vi "GasMeter3.vi"() -> ()   [LabVIEW 2012]
uses:
  <vilib>/DAQmx/read.llb/DAQmx Read (Analog 1D DBL NChan 1Samp).vi
panel:
  out "ANSI Placeholder 3":dbl
  out "Start Time ANSI 3":dbl
  out "ANSI Placeholder 2":dbl
  out "Start Time ANSI 2":dbl
  in  "Start ANSI 3":bool
  in  "HeatingValueLP 3":dbl=2450.0 min=2400.0 max=2600.0 step=5.0
  out "CF/HR 3":dbl format="%#_2g"
  out "HV 3":dbl
  out "Meter ID 3":dbl
  out "Gas 3":string
  in  "HeatingValueLP 2":dbl=2450.0 min=2400.0 max=2600.0 step=5.0
  in  "HeatingValueNG 2":dbl=990.0 min=990.0 max=1025.0 step=1.0
  out "Meter 6 Present":bool
  out "Meter 5 Present":bool
  out "Meter 4 Present":bool
  out "Meter 3 Present":bool
  out "Meter 2 Present":bool
  out "Meter 1 Present":bool
  out "Meter Type 6":string
  out "Meter Type 2":string
  out "Meter Type 4":string
  out "Meter Type 5":string
  out "Meter Type 3":string
  out "Meter Type 1":string
  out "Meter 6 Size":dbl
  out "Meter 5 Size":dbl
  out "Meter 4 Size":dbl
  out "Meter 3 Size":dbl
  out "Meter 2 Size":dbl
  out "Meter 1 Size":dbl
  out "ANSI Placeholder":dbl
  out "Start Time ANSI":dbl
  in  "Start ANSI":bool
  out "ANSI Average (BTU/hr)":dbl format="%#_5g"
  out "30 Second Average (BTU/hr)":dbl format="%#_5g"
  out "15 Second Average (BTU/hr)":dbl format="%#_5g"
  out "Reference6":dbl
  out "Reference5":dbl
  out "Reference4":dbl
  out "Reference3":dbl
  out "Reference2":dbl
  out "Reference1":dbl
  out "Time":dbl
  out "Num Record":dbl
  in  "HeatingValueLP":dbl=2450.0 min=2400.0 max=2600.0 step=5.0
  out "Output 6":dbl min=0.0 max=5.0 step=0.01
  out "Output 5":dbl min=0.0 max=5.0 step=0.01
  out "Output 4":dbl min=0.0 max=5.0 step=0.01
  out "Output 3":dbl min=0.0 max=5.0 step=0.01
  out "Output 2":dbl min=0.0 max=5.0 step=0.01
  out "Output 1":dbl min=0.0 max=5.0 step=0.01
  out "Signal":bool
  in  "Record":bool
  out "File Path":path
  out "CF/HR":dbl format="%#_2g"
  out "HV":dbl
  in  "HeatingValueNG":dbl=990.0 min=990.0 max=1025.0 step=1.0
  out "Meter ID":dbl
  out "Gas":string
  out "DisplayChart":cluster{"Flow Rate":dbl}(graph)
  out "Flow Rate":dbl format="%#_5g"
  # "STATION 1"
  # "STATION 3"
  # "Heating Value"
  # "Heating Value"
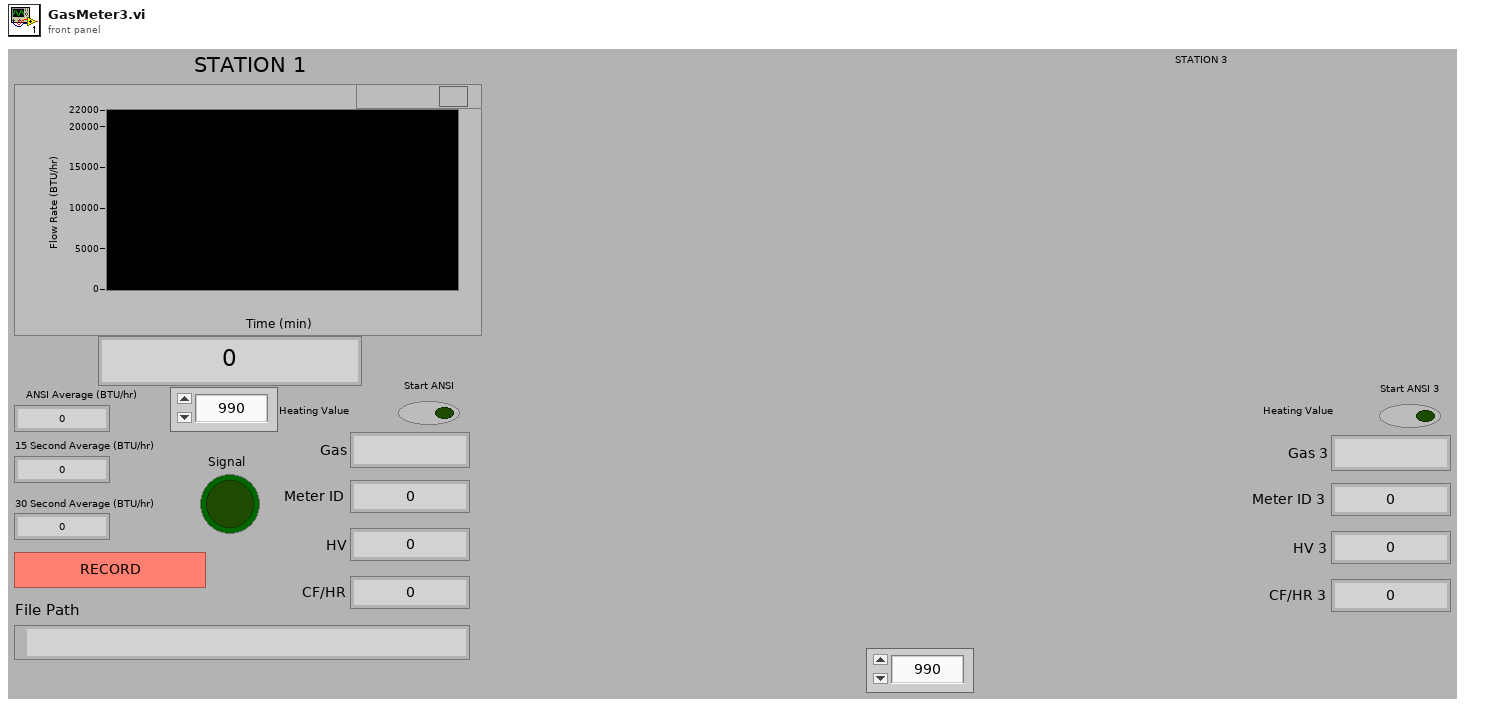
[diagram p1: front panel]
types:
  T1 = enum16{"open", "replace", "create", "open or create", "replace or create", "replace or create with confirmation"}
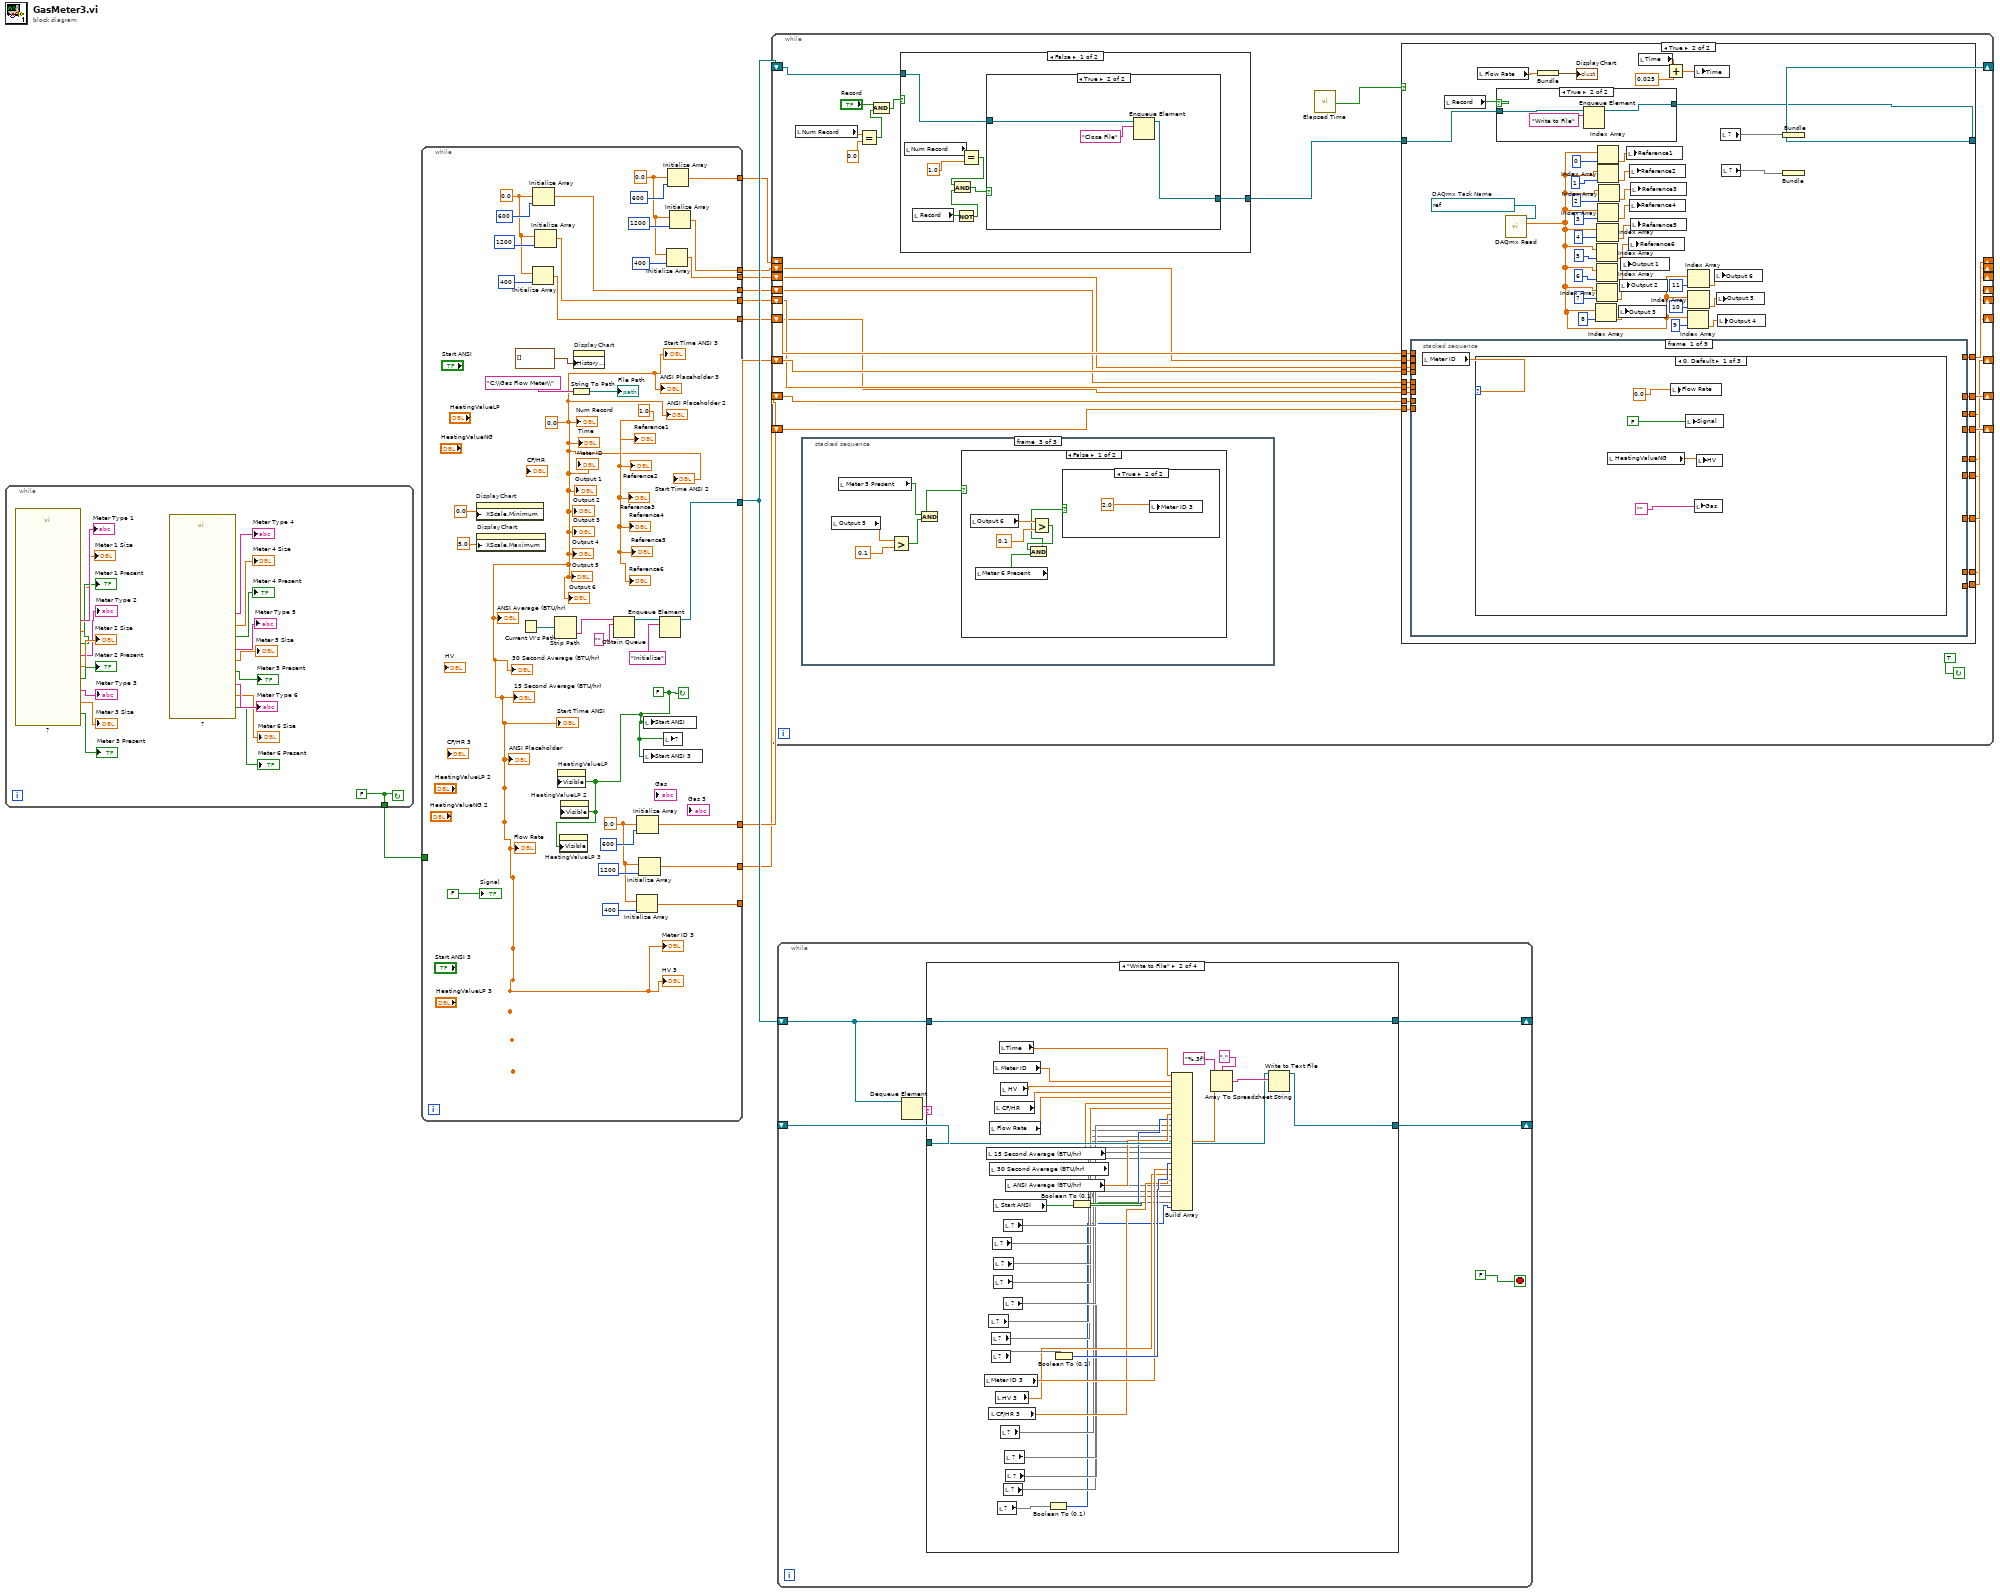
[diagram p0: block diagram]
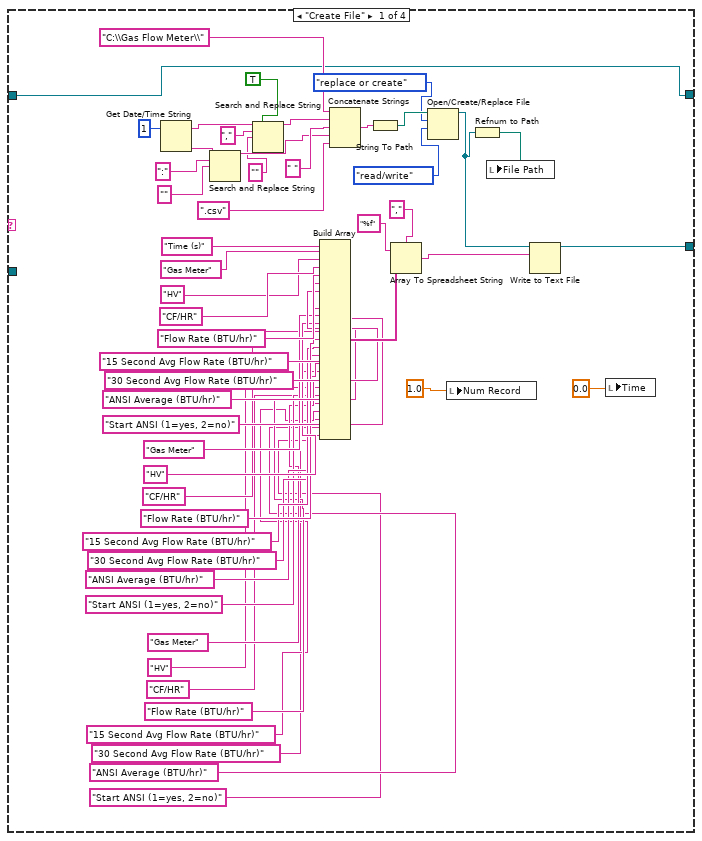
[diagram p2: hidden frame]
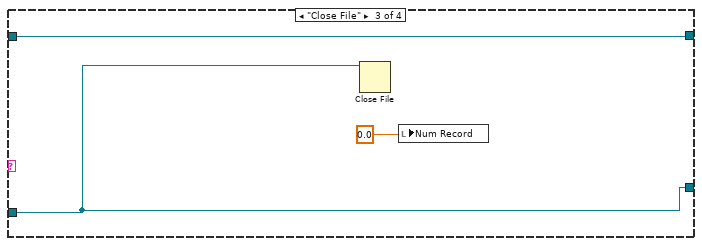
[diagram p3: hidden frame]
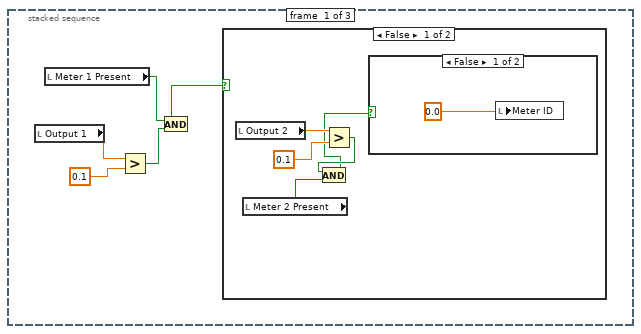
[diagram p5: hidden frame]
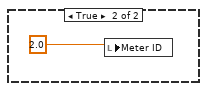
[diagram p6: hidden frame]
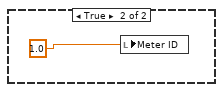
[diagram p7: hidden frame]
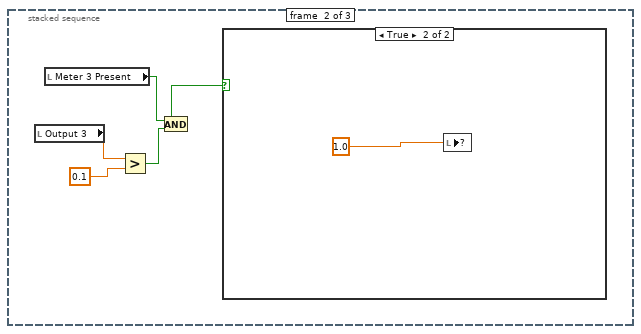
[diagram p8: hidden frame]
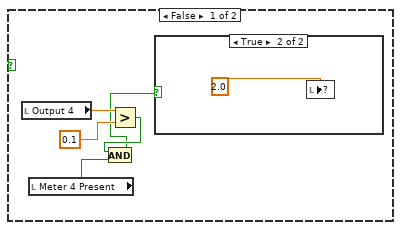
[diagram p9: hidden frame]
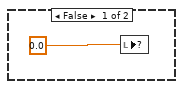
[diagram p10: hidden frame]
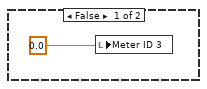
[diagram p11: hidden frame]
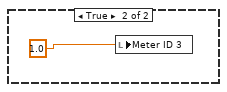
[diagram p12: hidden frame]
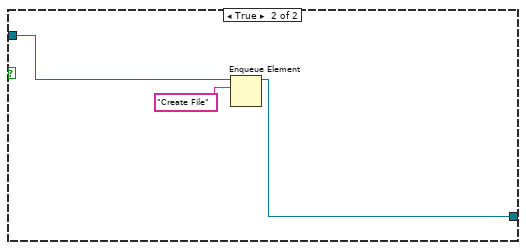
[diagram p14: hidden frame]
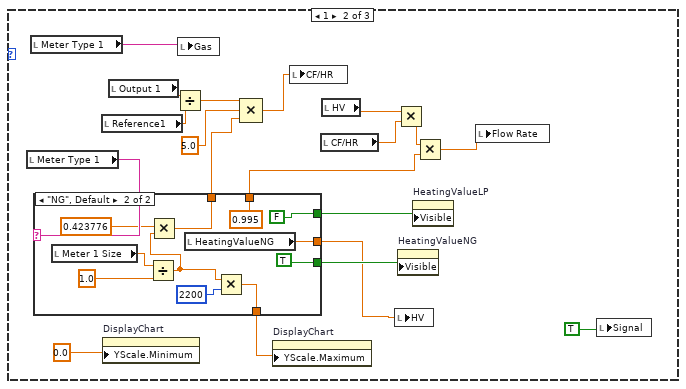
[diagram p16: hidden frame]
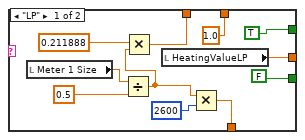
[diagram p17: hidden frame]
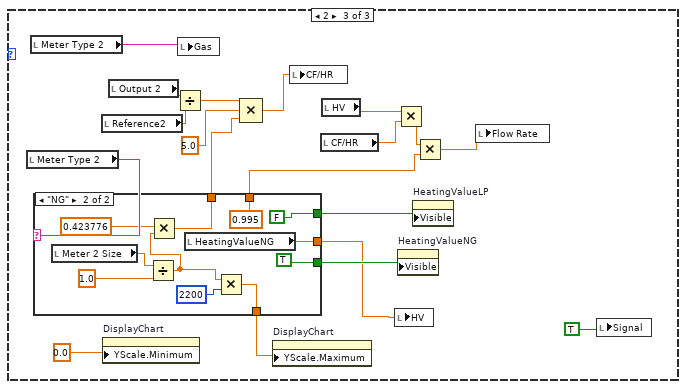
[diagram p18: hidden frame]
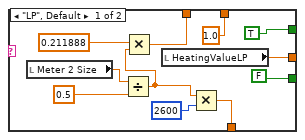
[diagram p19: hidden frame]
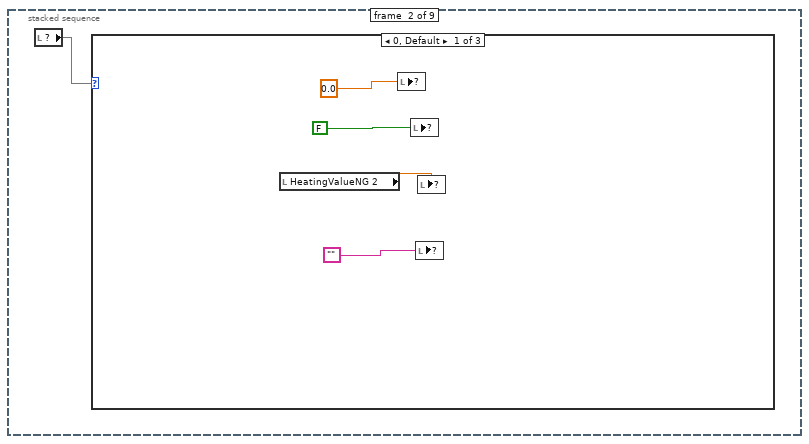
[diagram p20: hidden frame]
diagram:
  n1 = while {
    tunnel: [w29] -> w7
    stop <- w29 continue-if-true
    w29 = FALSE
    n2 = call "?"() -> ("Meter 3 Present?"=→"Meter 3 Present":bool, "Meter Size 3 (SLPM)"=→"Meter 3 Size":dbl, "Meter Type 3 (LP/NG)"=→"Meter Type 3":string, "Meter 2 Present?"=→"Meter 2 Present":bool, "Meter Size 2 (SLPM)"=→"Meter 2 Size":dbl, "Meter Type 2 (LP/NG)"=→"Meter Type 2":string, "Meter 1 Present?"=→"Meter 1 Present":bool, "Meter Size 1 (SLPM)"=→"Meter 1 Size":dbl, "Meter Type 1 (LP/NG)"=→"Meter Type 1":string)  [unwired: 9 in, 2 out]
    n3 = call "?"() -> ("Meter 6 Present?"=→"Meter 6 Present":bool, "Meter Size 6 (SLPM)"=→"Meter 6 Size":dbl, "Meter Type 6 (LP/NG)"=→"Meter Type 6":string, "Meter 5 Present?"=→"Meter 5 Present":bool, "Meter Size 5 (SLPM)"=→"Meter 5 Size":dbl, "Meter Type 5 (LP/NG)"=→"Meter Type 5":string, "Meter 4 Present?"=→"Meter 4 Present":bool, "Meter Size 4 (SLPM)"=→"Meter 4 Size":dbl, "Meter Type 4 (LP/NG)"=→"Meter Type 4":string)  [unwired: 9 in, 2 out]
  }
  n4 = while {
    tunnel: [w59] -> w11
    tunnel: [w55] -> w10
    tunnel: [w54] -> w9
    tunnel: [w51] -> w8
    tunnel: w7 -> [_]
    tunnel: [w46] -> w6
    tunnel: [w45] -> w5
    tunnel: [w44] -> w4
    tunnel: [w39] -> w3
    tunnel: [w38] -> w2
    tunnel: [w37] -> w1
    stop <- w34 continue-if-true
    w41 = 0.0
    w48 = 0.0
    w53 = 0.0
    w58 = 1.0
    w35 = 0.0
    w34 = FALSE
    n5 = property on="DisplayChart" class="WFChart (strict)"("XScale.Minimum"=0.0) -> ()  [unwired: 2 in, 2 out]
    n6 = property on="DisplayChart" class="WFChart (strict)"("XScale.Maximum"=5.0) -> ()  [unwired: 2 in, 2 out]
    n7 = Current VI's Path() -> (path=w64:path)
    n8 = Initialize Array(w41, 400) -> (w37:dbl[])
    n9 = Initialize Array(w41, 600) -> (w39:dbl[])
    n10 = Initialize Array(w41, 1200) -> (w38:dbl[])
    n11 = Strip Path(path=w64) -> (name=w62:string)  [unwired: 1 out]
    n12 = property on="HeatingValueLP" class="DigNum (strict)"("Visible"=w34) -> ()  [unwired: 2 in, 2 out]
    n13 = property on="HeatingValueLP 3" class="DigNum (strict)"("Visible"=w34) -> ()  [unwired: 2 in, 2 out]
    n14 = property on="HeatingValueLP 2" class="DigNum (strict)"("Visible"=w34) -> ()  [unwired: 2 in, 2 out]
    n15 = String To Path(string="C:\\Gas Flow Meter\\") -> (path=→"File Path":path)
    n16 = property on="DisplayChart" class="WFChart (strict)"("History Data"=cluster{"[0]":dbl}[] []) -> ()  [unwired: 2 in, 2 out]
    n17 = Obtain Queue(name (unnamed)=w62, element data type="") -> (queue out=w60:refnum<queue>)  [unwired: 3 in, 2 out]
    n18 = Initialize Array(w53, 400) -> (w51:dbl[])
    n19 = Initialize Array(w53, 600) -> (w55:dbl[])
    n20 = Initialize Array(w53, 1200) -> (w54:dbl[])
    n21 = local write "Start ANSI"(w34) -> ()
    n22 = local write "Start ANSI 3"(w34) -> ()
    n23 = Enqueue Element(queue=w60, element="Initialize") -> (queue out=w59:refnum<queue>)  [unwired: 2 in, 2 out]
    n24 = local write item#-1(w34) -> ()
    n25 = Initialize Array(w48, 400) -> (w44:dbl[])
    n26 = Initialize Array(w48, 600) -> (w46:dbl[])
    n27 = Initialize Array(w48, 1200) -> (w45:dbl[])
    "Num Record" <- w35
    "Time" <- w35
    "Meter ID" <- w35
    "Output 1" <- w35
    "Output 2" <- w35
    "Output 3" <- w35
    "Output 4" <- w35
    "Output 5" <- w35
    "Output 6" <- w35
    "Reference1" <- w58
    "Reference2" <- w58
    "Reference3" <- w58
    "Reference4" <- w58
    "Reference5" <- w58
    "Reference6" <- w58
    "30 Second Average (BTU/hr)" <- w35
    "15 Second Average (BTU/hr)" <- w35
    "ANSI Average (BTU/hr)" <- w35
    "Start Time ANSI" <- w35
    "ANSI Placeholder" <- w35
    "Flow Rate" <- w35
    "Signal" <- FALSE
    "Meter ID 3" <- w35
    "HV 3" <- w35
    "Start Time ANSI 3" <- w35
    "ANSI Placeholder 3" <- w35
    "ANSI Placeholder 2" <- w35
    "Start Time ANSI 2" <- w35
  }
  n28 = while {
    shift-right: [w92] -> _
    shift-left: w11 -> [w85]
    shift-right: [w91] -> _
    shift-left: w10 -> [w89]
    shift-right: [w90] -> _
    shift-left: w9 -> [w88]
    shift-right: [w87] -> _
    shift-left: w8 -> [w86]
    shift-right: [w77] -> _
    shift-left: w6 -> [w78]
    shift-right: [w75] -> _
    shift-left: w5 -> [w76]
    shift-right: [w73] -> _
    shift-left: w4 -> [w74]
    shift-right: [w71] -> _
    shift-left: w3 -> [w72]
    shift-right: [w69] -> _
    shift-left: w2 -> [w70]
    shift-right: [w67] -> _
    shift-left: w1 -> [w68]
    stop <- TRUE continue-if-true
    n29 = local read "Num Record"() -> (w81:dbl)
    n30 = stacked-sequence {
      frame #0 {
        n31 = local read "Output 1"() -> (w99:dbl)
        n32 = local read "Meter 1 Present"() -> (w96:bool)
        n33 = Greater?(x=w99, y=0.1) -> (0:w97:bool)
        n34 = And(x=w96, y=w97) -> (x .and. y?=w95:bool)
        n35 = case shown="False" w95 {
          frame False {
            n36 = local read "Output 2"() -> (w103:dbl)
            n37 = local read "Meter 2 Present"() -> (w102:bool)
            n38 = Greater?(x=w103, y=0.1) -> (0:w101:bool)
            n39 = And(x=w101, y=w102) -> (x .and. y?=w100:bool)
            n40 = case shown="False" w100 {
              frame False {
                n41 = local write "Meter ID"(0.0) -> ()
              }
              frame True {
                n42 = local write "Meter ID"(2.0) -> ()
              }
            }
          }
          frame True {
            n43 = local write "Meter ID"(1.0) -> ()
          }
        }
      }
      frame #1 {
        n44 = local read "Output 3"() -> (w112:dbl)
        n45 = local read "Meter 3 Present"() -> (w109:bool)
        n46 = Greater?(x=w112, y=0.1) -> (0:w110:bool)
        n47 = And(x=w109, y=w110) -> (x .and. y?=w108:bool)
        n48 = case shown="True" w108 {
          frame False {
            n49 = local read "Output 4"() -> (w116:dbl)
            n50 = local read "Meter 4 Present"() -> (w115:bool)
            n51 = Greater?(x=w116, y=0.1) -> (0:w114:bool)
            n52 = And(x=w114, y=w115) -> (x .and. y?=w113:bool)
            n53 = case shown="True" w113 {
              frame False {
                n54 = local write item#-1(0.0) -> ()
              }
              frame True {
                n55 = local write item#-1(2.0) -> ()
              }
            }
          }
          frame True {
            n56 = local write item#-1(1.0) -> ()
          }
        }
      }
      frame #2 {
        n57 = local read "Output 5"() -> (w125:dbl)
        n58 = local read "Meter 5 Present"() -> (w122:bool)
        n59 = Greater?(x=w125, y=0.1) -> (0:w123:bool)
        n60 = And(x=w122, y=w123) -> (x .and. y?=w121:bool)
        n61 = case shown="False" w121 {
          frame False {
            n62 = local read "Output 6"() -> (w129:dbl)
            n63 = local read "Meter 6 Present"() -> (w128:bool)
            n64 = Greater?(x=w129, y=0.1) -> (0:w127:bool)
            n65 = And(x=w127, y=w128) -> (x .and. y?=w126:bool)
            n66 = case shown="True" w126 {
              frame False {
                n67 = local write "Meter ID 3"(0.0) -> ()
              }
              frame True {
                n68 = local write "Meter ID 3"(2.0) -> ()
              }
            }
          }
          frame True {
            n69 = local write "Meter ID 3"(1.0) -> ()
          }
        }
      }
    }
    n70 = Equal?(x=w81, y=0.0) -> (x = y?=w80:bool)
    n71 = And(x="Record", y=w80) -> (x .and. y?=w79:bool)
    n72 = case shown="False" w79 {
      tunnel: w85 -> [w139 w147]
      tunnel: [w138 w146] -> w84
      frame False {
        n73 = local read "Num Record"() -> (w141:dbl)
        n74 = local read "Record"() -> (w135:bool)
        n75 = Not(x=w135) -> (.not. x?=w134:bool)
        n76 = Equal?(x=w141, y=1.0) -> (x = y?=w137:bool)
        n77 = And(x=w137, y=w134) -> (x .and. y?=w136:bool)
        n78 = case shown="True" w136 {
          tunnel: w139 -> [w142 w144]
          tunnel: [w142 w143] -> w138
          frame False {
          }
          frame True {
            n79 = Enqueue Element(queue=w144, element="Close File") -> (queue out=w143:refnum<queue>)  [unwired: 2 in, 2 out]
          }
        }
      }
      frame True {
        n80 = Enqueue Element(queue=w147, element="Create File") -> (queue out=w146:refnum<queue>)  [unwired: 2 in, 2 out]
      }
    }
    n81 = call "Elapsed Time"() -> ("Time has Elapsed"=w93:bool)  [unwired: 12 in, 7 out]
    n82 = case shown="True" w93 {
      tunnel: w84 -> [w158 w208]
      tunnel: [w158 w207] -> w92
      tunnel: w89 -> [w157 w180]
      tunnel: w88 -> [w156 w179]
      tunnel: [w157 w178] -> w91
      tunnel: [w156 w177] -> w90
      tunnel: w86 -> [w155 w176]
      tunnel: [w155 w175] -> w87
      tunnel: w78 -> [w152 w174]
      tunnel: [w152 w173] -> w77
      tunnel: w76 -> [w153 w172]
      tunnel: [w153 w171] -> w75
      tunnel: w74 -> [w154 w170]
      tunnel: [w154 w169] -> w73
      tunnel: w72 -> [w151 w168]
      tunnel: [w151 w167] -> w71
      tunnel: w70 -> [w150 w166]
      tunnel: [w150 w165] -> w69
      tunnel: w68 -> [w149 w164]
      tunnel: [w149 w163] -> w67
      frame False {
      }
      frame True {
        w206 = refnum<k21> "ReadFlowMeterIn"  # DAQmx Task Name
        n83 = stacked-sequence {
          tunnel: w180 -> [_ _ _ w500 _ _ _ _ _]
          tunnel: w179 -> [_ _ _ w499 _ _ _ _ _]
          tunnel: [_ _ _ w494 _ _ _ _ _] -> w178
          tunnel: [_ _ _ w490 _ _ _ _ _] -> w177
          tunnel: w176 -> [_ _ _ w484 _ _ _ _ _]
          tunnel: [_ _ _ w481 _ _ _ _ _] -> w175
          tunnel: w174 -> [_ _ _ _ w523 _ _ _ _]
          tunnel: [_ _ _ _ w510 _ _ _ _] -> w173
          tunnel: w172 -> [_ _ _ _ w517 _ _ _ _]
          tunnel: [_ _ _ _ w509 _ _ _ _] -> w171
          tunnel: w170 -> [_ _ _ _ w515 _ _ _ _]
          tunnel: [_ _ _ _ w508 _ _ _ _] -> w169
          tunnel: w168 -> [_ _ _ _ _ w544 _ _ _]
          tunnel: [_ _ _ _ _ w542 _ _ _] -> w167
          tunnel: w166 -> [_ _ _ _ _ w541 _ _ _]
          tunnel: [_ _ _ _ _ w539 _ _ _] -> w165
          tunnel: w164 -> [_ _ _ _ _ w538 _ _ _]
          tunnel: [_ _ _ _ _ w536 _ _ _] -> w163
          frame #0 {
            n84 = local read "Meter ID"() -> (w215:dbl)
            n85 = case shown="0, Default" w215 {
              frame 0, Default {
                n86 = local read "HeatingValueNG"() -> (w219:dbl)
                n87 = local write "Flow Rate"(0.0) -> ()
                n88 = local write "Signal"(FALSE) -> ()
                n89 = local write "Gas"("") -> ()
                n90 = local write "HV"(w219) -> ()
              }
              frame 1 {
                n91 = local read "Meter Type 1"() -> (w228:string)
                n92 = local read "Meter Type 1"() -> (w222:string)
                n93 = case shown="\"NG\", Default" w228 {
                  tunnel: [w246 w257] -> w227
                  tunnel: [TRUE FALSE] -> w226
                  tunnel: [FALSE TRUE] -> w225
                  tunnel: [1.0 0.995] -> w224
                  tunnel: [w240 w251] -> w223
                  tunnel: [w239 w250] -> w221
                  frame "LP" {
                    n94 = local read "Meter 1 Size"() -> (w248:dbl)
                    n95 = Divide(x=w248, y=0.5) -> (x/y=w241:dbl)
                    n96 = Multiply(x=0.211888, y=w241) -> (x*y=w246:dbl)
                    n97 = local read "HeatingValueLP"() -> (w239:dbl)
                    n98 = Multiply(x=w241, y=2600) -> (x*y=w240:dbl)
                  }
                  frame "NG", Default {
                    n99 = local read "Meter 1 Size"() -> (w259:dbl)
                    n100 = Divide(x=w259, y=1.0) -> (x/y=w252:dbl)
                    n101 = Multiply(x=0.423776, y=w252) -> (x*y=w257:dbl)
                    n102 = local read "HeatingValueNG"() -> (w250:dbl)
                    n103 = Multiply(x=w252, y=2200) -> (x*y=w251:dbl)
                  }
                }
                n104 = local read "Reference1"() -> (w232:dbl)
                n105 = property on="DisplayChart" class="WFChart (strict)"("YScale.Minimum"=0.0) -> ()  [unwired: 2 in, 2 out]
                n106 = local read "Output 1"() -> (w233:dbl)
                n107 = Divide(x=w233, y=w232) -> (x/y=w230:dbl)
                n108 = local write "Gas"(w222) -> ()
                n109 = Compound Arithmetic op=MULTIPLY(w230, 5.0, w227) -> (w220:dbl)
                n110 = property on="DisplayChart" class="WFChart (strict)"("YScale.Maximum"=w223) -> ()  [unwired: 2 in, 2 out]
                n111 = local write "CF/HR"(w220) -> ()
                n112 = local read "CF/HR"() -> (w235:dbl)
                n113 = local read "HV"() -> (w234:dbl)
                n114 = local write "HV"(w221) -> ()
                n115 = Multiply(x=w234, y=w235) -> (x*y=w236:dbl)
                n116 = property on="HeatingValueNG" class="DigNum (strict)"("Visible"=w225) -> ()  [unwired: 2 in, 2 out]
                n117 = property on="HeatingValueLP" class="DigNum (strict)"("Visible"=w226) -> ()  [unwired: 2 in, 2 out]
                n118 = Multiply(x=w236, y=w224) -> (x*y=w237:dbl)
                n119 = local write "Flow Rate"(w237) -> ()
                n120 = local write "Signal"(TRUE) -> ()
              }
              frame 2 {
                n121 = local read "Meter Type 2"() -> (w269:string)
                n122 = local read "Meter Type 2"() -> (w263:string)
                n123 = case shown="\"NG\"" w269 {
                  tunnel: [w287 w298] -> w268
                  tunnel: [TRUE FALSE] -> w267
                  tunnel: [FALSE TRUE] -> w266
                  tunnel: [1.0 0.995] -> w265
                  tunnel: [w281 w292] -> w264
                  tunnel: [w280 w291] -> w262
                  frame "LP", Default {
                    n124 = local read "Meter 2 Size"() -> (w289:dbl)
                    n125 = Divide(x=w289, y=0.5) -> (x/y=w282:dbl)
                    n126 = Multiply(x=0.211888, y=w282) -> (x*y=w287:dbl)
                    n127 = local read "HeatingValueLP"() -> (w280:dbl)
                    n128 = Multiply(x=w282, y=2600) -> (x*y=w281:dbl)
                  }
                  frame "NG" {
                    n129 = local read "Meter 2 Size"() -> (w300:dbl)
                    n130 = Divide(x=w300, y=1.0) -> (x/y=w293:dbl)
                    n131 = Multiply(x=0.423776, y=w293) -> (x*y=w298:dbl)
                    n132 = local read "HeatingValueNG"() -> (w291:dbl)
                    n133 = Multiply(x=w293, y=2200) -> (x*y=w292:dbl)
                  }
                }
                n134 = local read "Reference2"() -> (w273:dbl)
                n135 = property on="DisplayChart" class="WFChart (strict)"("YScale.Minimum"=0.0) -> ()  [unwired: 2 in, 2 out]
                n136 = local read "Output 2"() -> (w274:dbl)
                n137 = Divide(x=w274, y=w273) -> (x/y=w271:dbl)
                n138 = local write "Gas"(w263) -> ()
                n139 = Compound Arithmetic op=MULTIPLY(w271, 5.0, w268) -> (w261:dbl)
                n140 = property on="DisplayChart" class="WFChart (strict)"("YScale.Maximum"=w264) -> ()  [unwired: 2 in, 2 out]
                n141 = local write "CF/HR"(w261) -> ()
                n142 = local read "CF/HR"() -> (w276:dbl)
                n143 = local read "HV"() -> (w275:dbl)
                n144 = local write "HV"(w262) -> ()
                n145 = Multiply(x=w275, y=w276) -> (x*y=w277:dbl)
                n146 = property on="HeatingValueNG" class="DigNum (strict)"("Visible"=w266) -> ()  [unwired: 2 in, 2 out]
                n147 = property on="HeatingValueLP" class="DigNum (strict)"("Visible"=w267) -> ()  [unwired: 2 in, 2 out]
                n148 = Multiply(x=w277, y=w265) -> (x*y=w278:dbl)
                n149 = local write "Flow Rate"(w278) -> ()
                n150 = local write "Signal"(TRUE) -> ()
              }
            }
          }
          frame #1 {
            n151 = local read item#-1() -> (w302)
            n152 = case shown="0, Default" w302 {
              frame 0, Default {
                n153 = local read "HeatingValueNG 2"() -> (w306:dbl)
                n154 = local write item#-1(0.0) -> ()
                n155 = local write item#-1(FALSE) -> ()
                n156 = local write item#-1("") -> ()
                n157 = local write item#-1(w306) -> ()
              }
              frame 1 {
                w316 = 0.0
                n158 = local read "Meter Type 3"() -> (w315:string)
                n159 = local read "Meter Type 3"() -> (w309:string)
                n160 = case shown="\"LP\"" w315 {
                  tunnel: [w333 w344] -> w314
                  tunnel: [TRUE FALSE] -> w313
                  tunnel: [FALSE TRUE] -> w312
                  tunnel: [1.0 0.995] -> w311
                  tunnel: [w327 w338] -> w310
                  tunnel: [w326 w337] -> w308
                  frame "LP" {
                    n161 = local read "Meter 3 Size"() -> (w335:dbl)
                    n162 = Divide(x=w335, y=0.5) -> (x/y=w328:dbl)
                    n163 = Multiply(x=0.211888, y=w328) -> (x*y=w333:dbl)
                    n164 = local read "HeatingValueLP 2"() -> (w326:dbl)
                    n165 = Multiply(x=w328, y=2600) -> (x*y=w327:dbl)
                  }
                  frame "NG", Default {
                    n166 = local read "Meter 3 Size"() -> (w346:dbl)
                    n167 = Divide(x=w346, y=1.0) -> (x/y=w339:dbl)
                    n168 = Multiply(x=0.423776, y=w339) -> (x*y=w344:dbl)
                    n169 = local read "HeatingValueNG 2"() -> (w337:dbl)
                    n170 = Multiply(x=w339, y=2200) -> (x*y=w338:dbl)
                  }
                }
                n171 = local read "Reference3"() -> (w319:dbl)
                n172 = local read "Output 3"() -> (w320:dbl)
                n173 = Divide(x=w320, y=w319) -> (x/y=w317:dbl)
                n174 = local write item#-1(w309) -> ()
                n175 = Compound Arithmetic op=MULTIPLY(w317, 5.0, w314) -> (w307:dbl)
                n176 = local write item#-1(w307) -> ()
                n177 = local read item#-1() -> (w321)
                n178 = local read item#-1() -> (w322)
                n179 = Multiply(x=w321, y=w322) -> (x*y=w323:dbl)
                n180 = property on="HeatingValueNG 2" class="DigNum (strict)"("Visible"=w312) -> ()  [unwired: 2 in, 2 out]
                n181 = local write item#-1(w308) -> ()
                n182 = property on="HeatingValueLP 2" class="DigNum (strict)"("Visible"=w313) -> ()  [unwired: 2 in, 2 out]
                n183 = Multiply(x=w323, y=w311) -> (x*y=w324:dbl)
                n184 = local write item#-1(w324) -> ()
                n185 = local write item#-1(TRUE) -> ()
              }
              frame 2 {
                w357 = 0.0
                n186 = local read "Meter Type 4"() -> (w356:string)
                n187 = local read "Meter Type 4"() -> (w350:string)
                n188 = case shown="\"NG\", Default" w356 {
                  tunnel: [w374 w385] -> w355
                  tunnel: [TRUE FALSE] -> w354
                  tunnel: [FALSE TRUE] -> w353
                  tunnel: [1.0 0.995] -> w352
                  tunnel: [w368 w379] -> w351
                  tunnel: [w367 w378] -> w349
                  frame "LP" {
                    n189 = local read "Meter 4 Size"() -> (w376:dbl)
                    n190 = Divide(x=w376, y=0.5) -> (x/y=w369:dbl)
                    n191 = Multiply(x=0.211888, y=w369) -> (x*y=w374:dbl)
                    n192 = local read "HeatingValueLP 2"() -> (w367:dbl)
                    n193 = Multiply(x=w369, y=2600) -> (x*y=w368:dbl)
                  }
                  frame "NG", Default {
                    n194 = local read "Meter 4 Size"() -> (w387:dbl)
                    n195 = Divide(x=w387, y=1.0) -> (x/y=w380:dbl)
                    n196 = Multiply(x=0.423776, y=w380) -> (x*y=w385:dbl)
                    n197 = local read "HeatingValueNG 2"() -> (w378:dbl)
                    n198 = Multiply(x=w380, y=2200) -> (x*y=w379:dbl)
                  }
                }
                n199 = local read "Reference4"() -> (w360:dbl)
                n200 = local read "Output 4"() -> (w361:dbl)
                n201 = Divide(x=w361, y=w360) -> (x/y=w358:dbl)
                n202 = local write item#-1(w350) -> ()
                n203 = Compound Arithmetic op=MULTIPLY(w358, 5.0, w355) -> (w348:dbl)
                n204 = local write item#-1(w348) -> ()
                n205 = local read item#-1() -> (w362)
                n206 = local read item#-1() -> (w363)
                n207 = Multiply(x=w362, y=w363) -> (x*y=w364:dbl)
                n208 = property on="HeatingValueNG 2" class="DigNum (strict)"("Visible"=w353) -> ()  [unwired: 2 in, 2 out]
                n209 = local write item#-1(w349) -> ()
                n210 = property on="HeatingValueLP 2" class="DigNum (strict)"("Visible"=w354) -> ()  [unwired: 2 in, 2 out]
                n211 = Multiply(x=w364, y=w352) -> (x*y=w365:dbl)
                n212 = local write item#-1(w365) -> ()
                n213 = local write item#-1(TRUE) -> ()
              }
            }
          }
          frame #2 {
            n214 = local read "Meter ID 3"() -> (w389:dbl)
            n215 = case shown="0, Default" w389 {
              frame 0, Default {
                n216 = local read item#-1() -> (w393)
                n217 = local write item#-1(0.0) -> ()
                n218 = local write "Gas 3"("") -> ()
                n219 = local write "HV 3"(w393) -> ()
                n220 = local write item#-1(FALSE) -> ()
              }
              frame 1 {
                w403 = 0.0
                n221 = local read "Meter Type 5"() -> (w402:string)
                n222 = local read "Meter Type 5"() -> (w396:string)
                n223 = case shown="\"LP\"" w402 {
                  tunnel: [w420 w431] -> w401
                  tunnel: [TRUE FALSE] -> w400
                  tunnel: [FALSE TRUE] -> w399
                  tunnel: [1.0 0.995] -> w398
                  tunnel: [w414 w425] -> w397
                  tunnel: [w413 w424] -> w395
                  frame "LP" {
                    n224 = local read "Meter 5 Size"() -> (w422:dbl)
                    n225 = Divide(x=w422, y=0.5) -> (x/y=w415:dbl)
                    n226 = Multiply(x=0.211888, y=w415) -> (x*y=w420:dbl)
                    n227 = local read "HeatingValueLP 3"() -> (w413:dbl)
                    n228 = Multiply(x=w415, y=2600) -> (x*y=w414:dbl)
                  }
                  frame "NG", Default {
                    n229 = local read "Meter 5 Size"() -> (w433:dbl)
                    n230 = Divide(x=w433, y=1.0) -> (x/y=w426:dbl)
                    n231 = Multiply(x=0.423776, y=w426) -> (x*y=w431:dbl)
                    n232 = Multiply(x=w426, y=2200) -> (x*y=w425:dbl)
                    n233 = local read item#-1() -> (w424)
                  }
                }
                n234 = local read "Reference5"() -> (w406:dbl)
                n235 = local read "Output 5"() -> (w407:dbl)
                n236 = local write "Gas 3"(w396) -> ()
                n237 = Divide(x=w407, y=w406) -> (x/y=w404:dbl)
                n238 = Compound Arithmetic op=MULTIPLY(w404, 5.0, w401) -> (w394:dbl)
                n239 = local write "CF/HR 3"(w394) -> ()
                n240 = local read "CF/HR 3"() -> (w409:dbl)
                n241 = local read "HV 3"() -> (w408:dbl)
                n242 = local write "HV 3"(w395) -> ()
                n243 = Multiply(x=w408, y=w409) -> (x*y=w410:dbl)
                n244 = property on="HeatingValueLP 3" class="DigNum (strict)"("Visible"=w400) -> ()  [unwired: 2 in, 2 out]
                n245 = Multiply(x=w410, y=w398) -> (x*y=w411:dbl)
                n246 = local write item#-1(w411) -> ()
                n247 = local write item#-1(TRUE) -> ()
              }
              frame 2 {
                w444 = 0.0
                n248 = local read "Meter Type 6"() -> (w443:string)
                n249 = local read "Meter Type 6"() -> (w437:string)
                n250 = case shown="\"NG\", Default" w443 {
                  tunnel: [w461 w472] -> w442
                  tunnel: [TRUE FALSE] -> w441
                  tunnel: [FALSE TRUE] -> w440
                  tunnel: [1.0 0.995] -> w439
                  tunnel: [w455 w466] -> w438
                  tunnel: [w454 w465] -> w436
                  frame "LP" {
                    n251 = local read "Meter 6 Size"() -> (w463:dbl)
                    n252 = Divide(x=w463, y=0.5) -> (x/y=w456:dbl)
                    n253 = Multiply(x=0.211888, y=w456) -> (x*y=w461:dbl)
                    n254 = local read "HeatingValueLP 3"() -> (w454:dbl)
                    n255 = Multiply(x=w456, y=2600) -> (x*y=w455:dbl)
                  }
                  frame "NG", Default {
                    n256 = local read "Meter 6 Size"() -> (w474:dbl)
                    n257 = Divide(x=w474, y=1.0) -> (x/y=w467:dbl)
                    n258 = Multiply(x=0.423776, y=w467) -> (x*y=w472:dbl)
                    n259 = Multiply(x=w467, y=2200) -> (x*y=w466:dbl)
                    n260 = local read item#-1() -> (w465)
                  }
                }
                n261 = local read "Reference6"() -> (w447:dbl)
                n262 = local read "Output 6"() -> (w448:dbl)
                n263 = local write "Gas 3"(w437) -> ()
                n264 = Divide(x=w448, y=w447) -> (x/y=w445:dbl)
                n265 = Compound Arithmetic op=MULTIPLY(w445, 5.0, w442) -> (w435:dbl)
                n266 = local write "CF/HR 3"(w435) -> ()
                n267 = local read "CF/HR 3"() -> (w450:dbl)
                n268 = local read "HV 3"() -> (w449:dbl)
                n269 = local write "HV 3"(w436) -> ()
                n270 = Multiply(x=w449, y=w450) -> (x*y=w451:dbl)
                n271 = property on="HeatingValueLP 3" class="DigNum (strict)"("Visible"=w441) -> ()  [unwired: 2 in, 2 out]
                n272 = Multiply(x=w451, y=w439) -> (x*y=w452:dbl)
                n273 = local write item#-1(w452) -> ()
                n274 = local write item#-1(TRUE) -> ()
              }
            }
          }
          frame #3 {
            n275 = Delete From Array(array=w500, index=599) -> (array with subset deleted=w495:dbl[])  [unwired: 1 in, 1 out]
            n276 = Delete From Array(array=w484, index=399) -> (array with subset deleted=w482:dbl[])  [unwired: 1 in, 1 out]
            n277 = Delete From Array(array=w499, index=1199) -> (array with subset deleted=w496:dbl[])  [unwired: 1 in, 1 out]
            n278 = local read "Flow Rate"() -> (w477:dbl)
            n279 = Insert Into Array(array=w482, index=0, new element=w477) -> (w481:dbl[])
            n280 = Insert Into Array(array=w495, index=0, new element=w477) -> (w494:dbl[])
            n281 = Insert Into Array(array=w496, index=0, new element=w477) -> (w490:dbl[])
            n282 = Add Array Elements(numeric array=w481) -> (sum=w480:dbl)
            n283 = Array Size(array=w481) -> (size(s)=w479:i32)
            n284 = Add Array Elements(numeric array=w490) -> (sum=w489:dbl)
            n285 = Array Size(array=w490) -> (size(s)=w488:i32)
            n286 = Add Array Elements(numeric array=w494) -> (sum=w492:dbl)
            n287 = Array Size(array=w494) -> (size(s)=w493:i32)
            n288 = Divide(x=w480, y=w479) -> (x/y=w478:dbl)
            n289 = Divide(x=w489, y=w488) -> (x/y=w487:dbl)
            n290 = Divide(x=w492, y=w493) -> (x/y=w491:dbl)
            n291 = local write "15 Second Average (BTU/hr)"(w491) -> ()
            n292 = local write "ANSI Placeholder"(w478) -> ()
            n293 = local write "30 Second Average (BTU/hr)"(w487) -> ()
          }
          frame #4 {
            n294 = Delete From Array(array=w517, index=1199) -> (array with subset deleted=w516:dbl[])  [unwired: 1 in, 1 out]
            n295 = Delete From Array(array=w523, index=599) -> (array with subset deleted=w522:dbl[])  [unwired: 1 in, 1 out]
            n296 = Delete From Array(array=w515, index=399) -> (array with subset deleted=w514:dbl[])  [unwired: 1 in, 1 out]
            n297 = local read item#-1() -> (w504)
            n298 = Insert Into Array(array=w516, index=0, new element=w504) -> (w509:dbl[])
            n299 = Insert Into Array(array=w522, index=0, new element=w504) -> (w510:dbl[])
            n300 = Insert Into Array(array=w514, index=0, new element=w504) -> (w508:dbl[])
            n301 = Add Array Elements(numeric array=w509) -> (sum=w520:dbl)
            n302 = Array Size(array=w509) -> (size(s)=w521:i32)
            n303 = Add Array Elements(numeric array=w510) -> (sum=w524:dbl)
            n304 = Array Size(array=w510) -> (size(s)=w525:i32)
            n305 = Add Array Elements(numeric array=w508) -> (sum=w518:dbl)
            n306 = Array Size(array=w508) -> (size(s)=w519:i32)
            n307 = Divide(x=w520, y=w521) -> (x/y=w503:dbl)
            n308 = Divide(x=w524, y=w525) -> (x/y=w502:dbl)
            n309 = Divide(x=w518, y=w519) -> (x/y=w501:dbl)
            n310 = local write item#-1(w503) -> ()
            n311 = local write "ANSI Placeholder 2"(w501) -> ()
            n312 = local write item#-1(w502) -> ()
          }
          frame #5 {
            n313 = Delete From Array(array=w541, index=1199) -> (array with subset deleted=w540:dbl[])  [unwired: 1 in, 1 out]
            n314 = Delete From Array(array=w538, index=399) -> (array with subset deleted=w537:dbl[])  [unwired: 1 in, 1 out]
            n315 = Delete From Array(array=w544, index=599) -> (array with subset deleted=w543:dbl[])  [unwired: 1 in, 1 out]
            n316 = local read item#-1() -> (w535)
            n317 = Insert Into Array(array=w540, index=0, new element=w535) -> (w539:dbl[])
            n318 = Insert Into Array(array=w537, index=0, new element=w535) -> (w536:dbl[])
            n319 = Insert Into Array(array=w543, index=0, new element=w535) -> (w542:dbl[])
            n320 = Add Array Elements(numeric array=w539) -> (sum=w547:dbl)
            n321 = Add Array Elements(numeric array=w536) -> (sum=w545:dbl)
            n322 = Add Array Elements(numeric array=w542) -> (sum=w549:dbl)
            n323 = Array Size(array=w539) -> (size(s)=w548:i32)
            n324 = Array Size(array=w536) -> (size(s)=w546:i32)
            n325 = Array Size(array=w542) -> (size(s)=w550:i32)
            n326 = Divide(x=w547, y=w548) -> (x/y=w533:dbl)
            n327 = Divide(x=w545, y=w546) -> (x/y=w532:dbl)
            n328 = Divide(x=w549, y=w550) -> (x/y=w534:dbl)
            n329 = local write "ANSI Placeholder 3"(w532) -> ()
            n330 = local write item#-1(w533) -> ()
            n331 = local write item#-1(w534) -> ()
          }
          frame #6 {
            n332 = local read "Start ANSI"() -> (w551:bool)
            n333 = case shown="True" w551 {
              frame False {
              }
              frame True {
                n334 = local read "Start Time ANSI"() -> (w553:dbl)
                n335 = Equal?(x=w553, y=0.0) -> (x = y?=w552:bool)
                n336 = case shown="False" w552 {
                  frame False {
                    n337 = local read "Start Time ANSI"() -> (w559:dbl)
                    n338 = local read "Time"() -> (w556:dbl)
                    n339 = Add(x=w559, y=310) -> (x+y=w557:dbl)
                    n340 = Less Or Equal?(x=w556, y=w557) -> (x <= y?=w555:bool)
                    n341 = case shown="False" w555 {
                      frame False {
                        n342 = local read "ANSI Placeholder"() -> (w561:dbl)
                        n343 = local write "Start Time ANSI"(0.0) -> ()
                        n344 = local write "Start ANSI"(FALSE) -> ()
                        n345 = local write "ANSI Average (BTU/hr)"(w561) -> ()
                      }
                      frame True {
                      }
                    }
                  }
                  frame True {
                    n346 = local read "Time"() -> (w564:dbl)
                    n347 = local write "ANSI Average (BTU/hr)"(0.0) -> ()
                    n348 = local write "Start Time ANSI"(w564) -> ()
                  }
                }
              }
            }
          }
          frame #7 {
            n349 = local read item#-1() -> (w565)
            n350 = case shown="True" w565 {
              frame False {
              }
              frame True {
                n351 = local read "Start Time ANSI 2"() -> (w567:dbl)
                n352 = Equal?(x=w567, y=0.0) -> (x = y?=w566:bool)
                n353 = case shown="False" w566 {
                  frame False {
                    n354 = local read "Start Time ANSI 2"() -> (w573:dbl)
                    n355 = local read "Time"() -> (w570:dbl)
                    n356 = Add(x=w573, y=310) -> (x+y=w571:dbl)
                    n357 = Less Or Equal?(x=w570, y=w571) -> (x <= y?=w569:bool)
                    n358 = case shown="False" w569 {
                      frame False {
                        n359 = local read "ANSI Placeholder 2"() -> (w575:dbl)
                        n360 = local write "Start Time ANSI 2"(0.0) -> ()
                        n361 = local write item#-1(FALSE) -> ()
                        n362 = local write item#-1(w575) -> ()
                      }
                      frame True {
                      }
                    }
                  }
                  frame True {
                    n363 = local read "Time"() -> (w578:dbl)
                    n364 = local write "Start Time ANSI 2"(w578) -> ()
                    n365 = local write item#-1(0.0) -> ()
                  }
                }
              }
            }
          }
          frame #8 {
            n366 = local read "Start ANSI 3"() -> (w579:bool)
            n367 = case shown="True" w579 {
              frame False {
              }
              frame True {
                n368 = local read "Start Time ANSI 3"() -> (w581:dbl)
                n369 = Equal?(x=w581, y=0.0) -> (x = y?=w580:bool)
                n370 = case shown="False" w580 {
                  frame False {
                    n371 = local read "Start Time ANSI 3"() -> (w587:dbl)
                    n372 = local read "Time"() -> (w584:dbl)
                    n373 = Add(x=w587, y=310) -> (x+y=w585:dbl)
                    n374 = Less Or Equal?(x=w584, y=w585) -> (x <= y?=w583:bool)
                    n375 = case shown="False" w583 {
                      frame False {
                        n376 = local read "ANSI Placeholder 3"() -> (w589:dbl)
                        n377 = local write "Start Time ANSI 3"(0.0) -> ()
                        n378 = local write "Start ANSI 3"(FALSE) -> ()
                        n379 = local write item#-1(w589) -> ()
                      }
                      frame True {
                      }
                    }
                  }
                  frame True {
                    n380 = local read "Time"() -> (w592:dbl)
                    n381 = local write "Start Time ANSI 3"(w592) -> ()
                    n382 = local write item#-1(0.0) -> ()
                  }
                }
              }
            }
          }
        }
        n383 = local read "Record"() -> (w212:bool)
        n384 = local read "Flow Rate"() -> (w214:dbl)
        n385 = case shown="True" w212 {
          tunnel: w208 -> [w593 w595]
          tunnel: [w593 w594] -> w207
          frame False {
          }
          frame True {
            n386 = Enqueue Element(queue=w595, element="Write to File") -> (queue out=w594:refnum<queue>)  [unwired: 2 in, 2 out]
          }
        }
        n387 = call-poly <vilib>:"DAQmx Read.vi"("task/channels in"=w206) -> ("data"=w205:dbl[])  [unwired: 12 in, 2 out]
        n388 = Bundle("Flow Rate"=w214) -> (→"DisplayChart":cluster{"Flow Rate":dbl})  [unwired: 1 in]
        n389 = Index Array(array=w205, index=8) -> (element=w189:dbl)
        n390 = Index Array(array=w205, index=5) -> (element=w186:dbl)
        n391 = Index Array(array=w205, index=6) -> (element=w187:dbl)
        n392 = Index Array(array=w205, index=7) -> (element=w188:dbl)
        n393 = Index Array(array=w205, index=4) -> (element=w185:dbl)
        n394 = Index Array(array=w205, index=0) -> (element=w181:dbl)
        n395 = Index Array(array=w205, index=1) -> (element=w182:dbl)
        n396 = Index Array(array=w205, index=3) -> (element=w184:dbl)
        n397 = Index Array(array=w205, index=2) -> (element=w183:dbl)
        n398 = local write "Output 3"(w189) -> ()
        n399 = local write "Output 2"(w188) -> ()
        n400 = local write "Output 1"(w187) -> ()
        n401 = local write "Reference1"(w181) -> ()
        n402 = local write "Reference6"(w186) -> ()
        n403 = local write "Reference2"(w182) -> ()
        n404 = local write "Reference4"(w184) -> ()
        n405 = local write "Reference3"(w183) -> ()
        n406 = local write "Reference5"(w185) -> ()
        n407 = local read "Time"() -> (w210:dbl)
        n408 = Add(x=w210, y=0.025) -> (x+y=w209:dbl)
        n409 = Index Array(array=w205, index=9) -> (element=w190:dbl)
        n410 = Index Array(array=w205, index=11) -> (element=w192:dbl)
        n411 = Index Array(array=w205, index=10) -> (element=w191:dbl)
        n412 = local write "Time"(w209) -> ()
        n413 = local write "Output 6"(w192) -> ()
        n414 = local write "Output 5"(w191) -> ()
        n415 = local write "Output 4"(w190) -> ()
        n416 = local read item#-1() -> (w162)
        n417 = local read item#-1() -> (w161)
        n418 = Bundle(w162) -> (w160:cluster{void})  [unwired: 1 in]
        n419 = Bundle(w161) -> (w159:cluster{void})  [unwired: 1 in]
      }
    }
  }
  n420 = while {
    shift-right: [w600] -> _
    shift-left: w11 -> [w597]
    shift-right: [w599] -> _
    shift-left: _ -> [w598]
    stop <- FALSE stop-if-true
    n421 = Dequeue Element(queue=w597) -> (element=w601:string)  [unwired: 2 in, 3 out]
    n422 = case shown="\"Write to File\"" w601 {
      tunnel: [w624 w680 w691 w694] -> w600
      tunnel: w597 -> [w624 w680 w691 w694]
      tunnel: [w623 w678 w690 w693] -> w599
      tunnel: w598 -> [_ w679 w690 w693]
      frame "Create File" {
        n423 = Get Date/Time String(date format (0)=1) -> (date string=w629:string, time string=w626:string)  [unwired: 2 in]
        n424 = Search and Replace String(input string=w626, search string=":", replace string="") -> (result string=w635:string)  [unwired: 5 in, 3 out]
        n425 = Search and Replace String(replace all?=TRUE, input string=w629, search string=",", replace string="") -> (result string=w636:string)  [unwired: 4 in, 3 out]
        n426 = Build Array("Time (s)", "Gas Meter", "HV", "CF/HR", "Flow Rate (BTU/hr)", "15 Second Avg Flow Rate (BTU/hr)", "30 Second Avg Flow Rate (BTU/hr)", "ANSI Average (BTU/hr)", "Start ANSI (1=yes, 2=no)", "Gas Meter", "HV", "CF/HR", "Flow Rate (BTU/hr)", "15 Second Avg Flow Rate (BTU/hr)", "30 Second Avg Flow Rate (BTU/hr)", "ANSI Average (BTU/hr)", "Start ANSI (1=yes, 2=no)", "Gas Meter", "HV", "CF/HR", "Flow Rate (BTU/hr)", "15 Second Avg Flow Rate (BTU/hr)", "30 Second Avg Flow Rate (BTU/hr)", "ANSI Average (BTU/hr)", "Start ANSI (1=yes, 2=no)") -> (w646:string[])
        n427 = Concatenate Strings("C:\\Gas Flow Meter\\", w636, " ", w635, ".csv") -> (w632:string)
        n428 = String To Path(string=w632) -> (path=w652:path)
        n429 = Array To Spreadsheet String(delimiter (Tab)=",", array=w646, 3:"%f" ("format string")) -> (spreadsheet string=w647:string)
        n430 = Open/Create/Replace File(file path (use dialog)=w652, operation (0:open)=T1."replace or create", access (0:read/write)=enum16{"read/write", "read-only", "write-only"}."read/write") -> (refnum out=w654:refnum<file>)  [unwired: 3 in, 2 out]
        n431 = local write "Num Record"(1.0) -> ()
        n432 = Refnum to Path(1:w654) -> (0:w653:path)
        n433 = local write "File Path"(w653) -> ()
        n434 = Write to Text File(file (use dialog)=w654, text=w647) -> (refnum out=w623:refnum<file>)  [unwired: 2 in, 2 out]
        n435 = local write "Time"(0.0) -> ()
      }
      frame "Write to File" {
        n436 = local read "Meter ID 3"() -> (w662:dbl)
        n437 = local read "15 Second Average (BTU/hr)"() -> (w676:dbl)
        n438 = local read item#-1() -> (w665)
        n439 = local read "CF/HR 3"() -> (w660:dbl)
        n440 = local read "Flow Rate"() -> (w683:dbl)
        n441 = local read "30 Second Average (BTU/hr)"() -> (w677:dbl)
        n442 = local read item#-1() -> (w664)
        n443 = local read item#-1() -> (w671)
        n444 = local read item#-1() -> (w669)
        n445 = local read item#-1() -> (w667)
        n446 = local read "Meter ID"() -> (w686:dbl)
        n447 = local read "Start ANSI"() -> (w674:bool)
        n448 = local read item#-1() -> (w668)
        n449 = local read "CF/HR"() -> (w684:dbl)
        n450 = local read "HV 3"() -> (w661:dbl)
        n451 = local read item#-1() -> (w672)
        n452 = local read "Time"() -> (w687:dbl)
        n453 = local read item#-1() -> (w659)
        n454 = local read "HV"() -> (w685:dbl)
        n455 = local read item#-1() -> (w670)
        n456 = local read item#-1() -> (w666)
        n457 = local read item#-1() -> (w656)
        n458 = local read item#-1() -> (w658)
        n459 = local read "ANSI Average (BTU/hr)"() -> (w675:dbl)
        n460 = local read item#-1() -> (w657)
        n461 = Boolean To (0,1)(Boolean=w672) -> (0, 1=w655:i16)
        n462 = Boolean To (0,1)(Boolean=w671) -> (0, 1=w663:i16)
        n463 = Boolean To (0,1)(Boolean=w674) -> (0, 1=w673:i16)
        n464 = Build Array(w687, w686, w685, w684, w683, w676, w677, w675, w673, w670, w669, w668, w667, w666, w665, w664, w663, w662, w661, w660, w659, w658, w657, w656, w655) -> (w682:dbl[])
        n465 = Array To Spreadsheet String(delimiter (Tab)=",", array=w682, 3:"%.3f" ("format string")) -> (spreadsheet string=w681:string)
        n466 = Write to Text File(file (use dialog)=w679, text=w681) -> (refnum out=w678:refnum<file>)  [unwired: 2 in, 2 out]
      }
      frame "Close File" {
        n467 = Close File(refnum=w690) -> ()  [unwired: 1 in, 2 out]
        n468 = local write "Num Record"(0.0) -> ()
      }
      frame "Initialize", Default {
      }
    }
  }
